vi "LoadVI.vi"(1 "Path":string) -> (0 "VI":refnum<vi>)   [LabVIEW 2014]
uses:
  VI.global.vi
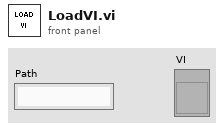
[diagram p1: front panel]
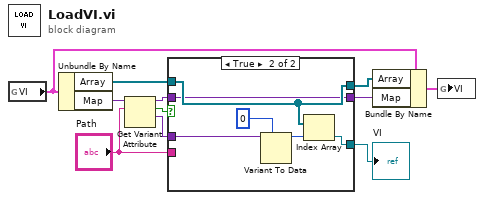
[diagram p0: block diagram]
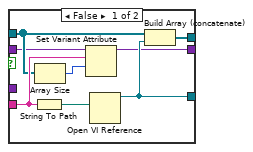
[diagram p2: hidden frame]
diagram:
  n1 = global read "VI.global.vi" "VI"() -> (w9:cluster{"Array":refnum<vi>[], "Map":variant})
  n2 = Unbundle By Name(w9) -> ("Array"=w11:refnum<vi>[], "Map"=w2:variant)
  n3 = Get Variant Attribute(Variant=w2, name="Path") -> (duplicate Variant=w5:variant, found=w6:bool, value=w3:variant)  [unwired: 2 in, 1 out]
  n4 = case shown="True" w6 {
    tunnel: "Path" -> [w19 _]
    tunnel: w3 -> [_ w25]
    tunnel: w5 -> [w13 w20]
    tunnel: [w16 w22] -> w7
    tunnel: w11 -> [w14 w21]
    tunnel: [w15 w21] -> w10
    tunnel: [w12 w20] -> w1
    frame False {
      n5 = String To Path(string=w19) -> (path=w18:path)
      n6 = Array Size(array=w14) -> (size(s)=w17:i32)
      n7 = Set Variant Attribute(Variant=w13, name=w19, value=w17) -> (Variant out=w12:variant)  [unwired: 1 in, 2 out]
      n8 = Open VI Reference(vi path=w18) -> (vi reference=w16:refnum<vi>)  [unwired: 5 in, 1 out]
      n9 = Build Array (concatenate)(w14, w16) -> (w15:refnum<vi>[])
    }
    frame True {
      n10 = Variant To Data(type=0 ("index"), Variant=w25) -> (data=w23:i32)  [unwired: 1 in, 1 out]
      n11 = Index Array(array=w21, index=w23) -> (element=w22:refnum<vi>)
    }
  }
  "VI" <- w7
  n12 = Bundle By Name(cluster=w9, "Array"=w10, "Map"=w1) -> (w8:cluster{"Array":refnum<vi>[], "Map":variant})
  n13 = global write "VI.global.vi" "VI"(w8) -> ()
